vi "10ms loop.vi"(6 "i":i32=12773, 8 "Potent":T2, 9 "Arm Angle":T2={"DevStatus"={"status"=FALSE, "code"=0, "source"=""}, "Analog Module"=enum."Analog Module 1", "Analog Channel"=enum."AI 2"}, 10 "Shooter":T5={"Device"=enum."USB 2"}, 11 "Driver":T5) -> ()   [LabVIEW 2012]
uses:
  <vilib>/Rock Robotics/WPI/AnalogChannel/WPI_AnalogChannelDevRef.ctl
  <vilib>/Rock Robotics/SystemInterfaces/Typedef/FPGA_TypedefAnalogModule.ctl
  <vilib>/Rock Robotics/SystemInterfaces/AI/FPGA_AIChannel.ctl
  <vilib>/Rock Robotics/WPI/Joystick/WPI_JoystickDevRef.ctl
  <vilib>/Rock Robotics/WPI/Joystick/WPI_JoystickDeviceEnum.ctl
  Robot Global Data.vi
panel:
  out "Shooter":T1={"axis 1 (x)"=-0.03937007874015748, "axis 2 (y)"=-0.05511811023622047, "axis 3 (throttle)"=-1.0, "axis 4"=0.0, "axis 5"=0.0, "axis 6"=0.0}
  out "Loop Count":i32=12774
  out "Arm Angle":dbl=1.8048920990000001
  in  "Shooter":dbl(slide)=0.55 min=0.0 max=1.0 step=0.01 scale=0.0..1.0 scale format="%#_2g"
  out "Voltage":dbl=4.728436393
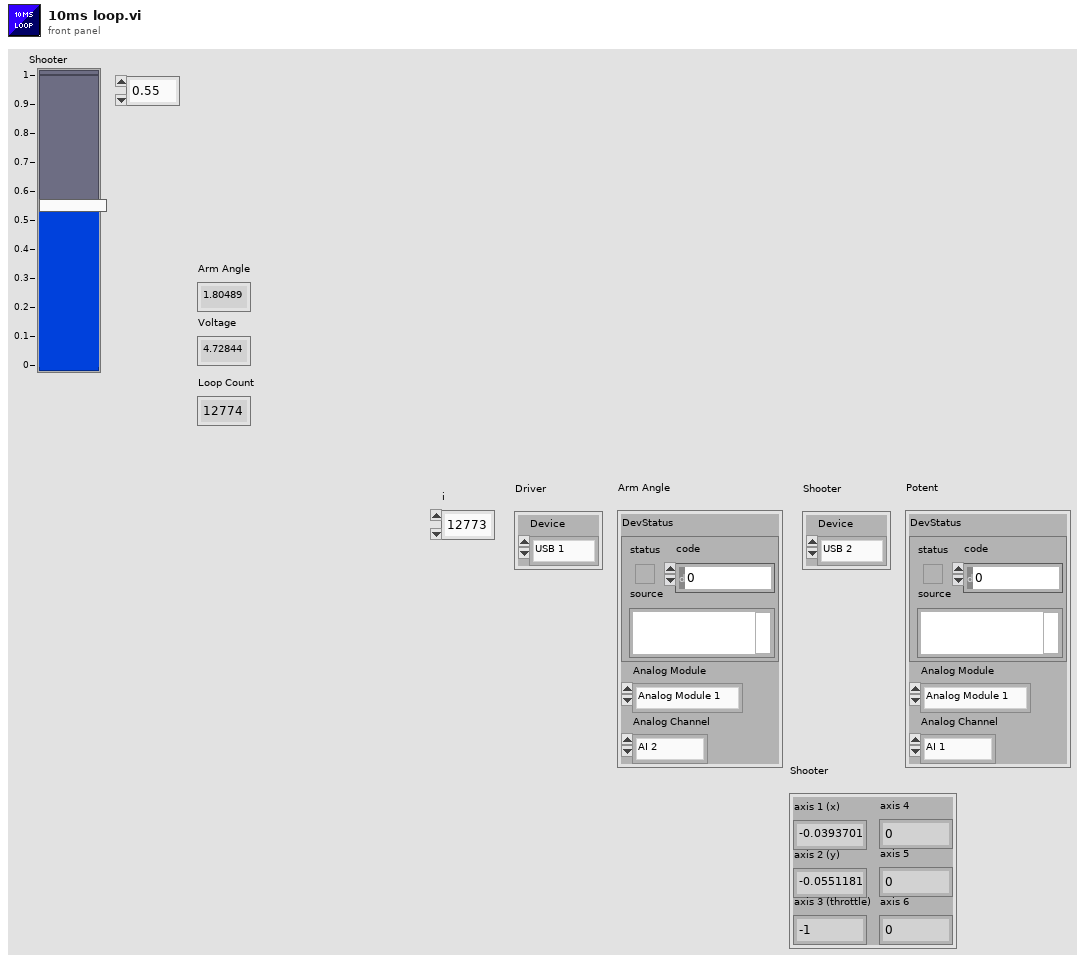
[diagram p1: front panel]
types:
  T1 = cluster{"axis 1 (x)":dbl, "axis 2 (y)":dbl, "axis 3 (throttle)":dbl, "axis 4":dbl, "axis 5":dbl, "axis 6":dbl}
  T2 = typedef "WPI_AnalogChannelDevRef.ctl" = cluster{"DevStatus":errorcluster, "Analog Module":T3, "Analog Channel":T4}
  T3 = typedef "FPGA_TypedefAnalogModule.ctl" = enum16{"Analog Module 1", "Analog Module 2"}
  T4 = typedef "FPGA_AIChannel.ctl" = enum8{"AI 1", "AI 2", "AI 3", "AI 4", "AI 5", "AI 6", "AI 7", "AI 8", "Invalid"}
  T5 = typedef "WPI_JoystickDevRef.ctl" = cluster{"Device":T6}
  T6 = typedef "WPI_JoystickDeviceEnum.ctl" = enum16{"USB 1", "USB 2", "USB 3", "USB 4", "Kinect 1", "Kinect 2"}
  T7 = typedef "WPI_JoystickButtonState.ctl" = cluster{"Button 1":bool, "Button 2":bool, "Button 3":bool, "Button 4":bool, "Button 5":bool, "Button 6":bool, "Button 7":bool, "Button 8":bool, "Button 9":bool, "Button 10":bool, "Button 11":bool, "Button 12":bool}
  T8 = cluster{"Button 6":bool, "Button 7":bool, "Button 11":bool, "Button 10":bool, "Button 2":bool, "Button 3":bool, "Button 1":bool, "Button 4":bool}
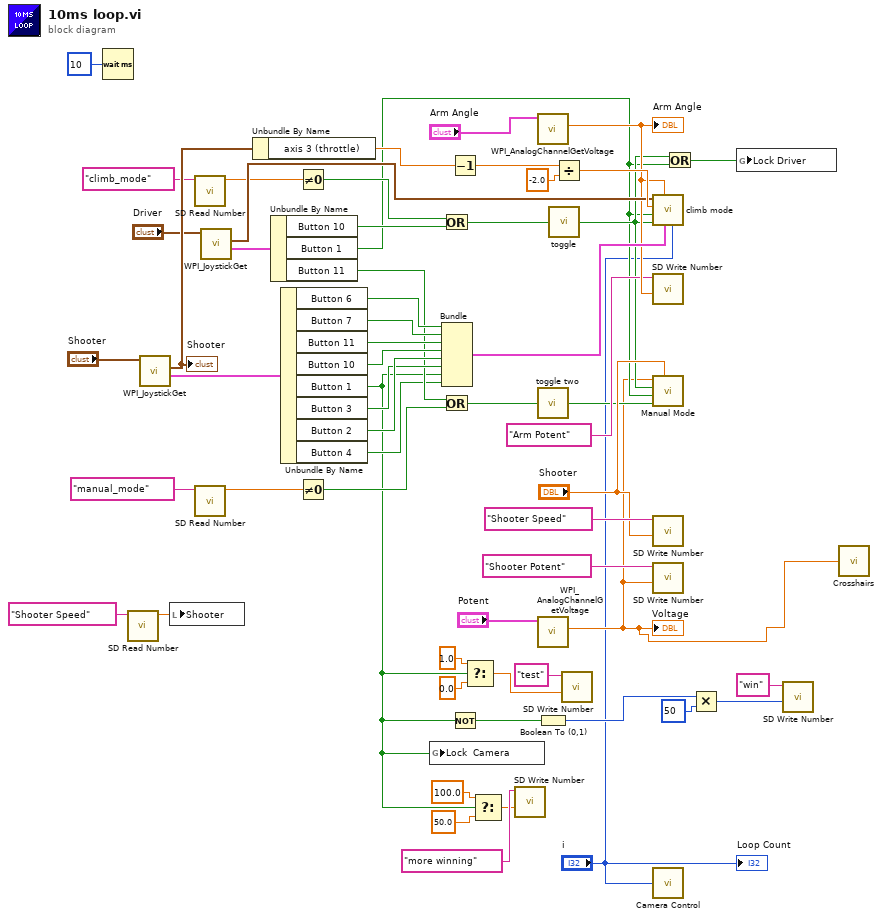
[diagram p0: block diagram]
diagram:
  n1 = Wait (ms)(milliseconds to wait=u32 10) -> ()  [unwired: 1 out]
  n2 = call <vilib>:"SD Read Number.vi"("Name"="Shooter Speed") -> ("Numeric"=w2:dbl)  [unwired: 8 in, 2 out]
  n3 = call <vilib>:"WPI_JoystickGet.vi"("JoystickDevRef"="Shooter") -> ("Buttons"=w56:T7, "Axes"=w50:T1)  [unwired: 4 in, 1 out]
  "Shooter" <- w50
  n4 = local write "Shooter"(w2) -> ()
  n5 = call <vilib>:"SD Read Number.vi"("Name"="climb_mode") -> ("Numeric"=w33:dbl)  [unwired: 8 in, 2 out]
  n6 = call <vilib>:"SD Read Number.vi"("Name"="manual_mode") -> ("Numeric"=w32:dbl)  [unwired: 8 in, 2 out]
  n7 = call <vilib>:"WPI_JoystickGet.vi"("JoystickDevRef"="Driver") -> ("Buttons"=w57:T7, "Axes"=w43:T1)  [unwired: 4 in, 1 out]
  n8 = Unbundle By Name(w50) -> ("axis 3 (throttle)"=w47:dbl)
  n9 = Unbundle By Name(w57) -> ("Button 10"=w29:bool, "Button 1"=w5:bool, "Button 11"=w26:bool)
  n10 = Unbundle By Name(w56) -> ("Button 6"=w54:bool, "Button 7"=w53:bool, "Button 11"=w52:bool, "Button 10"=w51:bool, "Button 1"=w11:bool, "Button 3"=w45:bool, "Button 2"=w46:bool, "Button 4"=w20:bool)
  n11 = Not Equal To 0?(x=w33) -> (x != 0?=w34:bool)
  n12 = Not Equal To 0?(x=w32) -> (x != 0?=w27:bool)
  n13 = global write "Robot Global Data.vi" "Lock  Camera"(w11) -> ()
  n14 = Or(x=w34, y=w29) -> (x .or. y?=w28:bool)
  n15 = Bundle("Button 6"=w54, "Button 7"=w53, "Button 11"=w52, "Button 10"=w51, "Button 2"=w46, "Button 3"=w45, "Button 1"=w11, "Button 4"=w20) -> (w19:T8)  [unwired: 1 in]
  n16 = Or(x=w26, y=w27) -> (x .or. y?=w25:bool)
  n17 = Decrement(x=w47) -> (x-1=w48:dbl)
  n18 = Not(x=w11) -> (.not. x?=w39:bool)
  n19 = Select(t=1.0, s=w11, f=0.0) -> (s? t:f=w23:dbl)
  n20 = Select(t=100.0, s=w11, f=50.0) -> (s? t:f=w12:dbl)
  n21 = call <vilib>:"SD Write Number.vi"("Numeric"=w12, "Name"="more winning") -> ()  [unwired: 8 in, 2 out]
  n22 = call <vilib>:"WPI_AnalogChannelGetVoltage.vi"("AIDeviceRef"="Arm Angle") -> ("Voltage"=w16:dbl)  [unwired: 8 in, 2 out]
  "Arm Angle" <- w16
  n23 = call "toggle two.vi"("Button In"=w25) -> ("tggle Out"=w6:bool)
  n24 = call <vilib>:"WPI_AnalogChannelGetVoltage.vi"("AIDeviceRef"="Potent") -> ("Voltage"=w4:dbl)  [unwired: 8 in, 2 out]
  "Voltage" <- w4
  n25 = Boolean To (0,1)(Boolean=w39) -> (0, 1=w13:i16)
  n26 = call "toggle.vi"("Btn In"=w28) -> ("Toggle Out"=w7:bool)
  n27 = Divide(x=w48, y=-2.0) -> (x/y=w44:dbl)
  n28 = call <vilib>:"SD Write Number.vi"("Numeric"=w23, "Name"="test") -> ()  [unwired: 8 in, 2 out]
  n29 = call "climb mode.vi"("i"="i", "Joystick 2"=w19, "Arm Angle"=w16, "engage climb"=w7, "Button 1"=w5, "Slide"=w44, "Joystick 1 Axes"=w43) -> ()  [unwired: 5 in]
  n30 = call <vilib>:"SD Write Number.vi"("Numeric"=w16, "Name"="Arm Potent") -> ()  [unwired: 8 in, 2 out]
  n31 = call "Manual Mode.vi"("potent"=w4, "Shooter"="Shooter", "climb"=w7, "Button 1"=w5, "manual"=w6) -> ()  [unwired: 4 in]
  n32 = call <vilib>:"SD Write Number.vi"("Numeric"="Shooter", "Name"="Shooter Speed") -> ()  [unwired: 8 in, 2 out]
  n33 = call <vilib>:"SD Write Number.vi"("Numeric"=w4, "Name"="Shooter Potent") -> ()  [unwired: 8 in, 2 out]
  n34 = call "Camera Control.vi"("i"="i") -> ()  [unwired: 1 in]
  n35 = Or(x=w7, y=w5) -> (x .or. y?=w55:bool)
  n36 = Multiply(x=w13, y=i16 50) -> (x*y=w41:i16)
  n37 = global write "Robot Global Data.vi" "Lock Driver"(w55) -> ()
  n38 = call <vilib>:"SD Write Number.vi"("Numeric"=w41, "Name"="win") -> ()  [unwired: 8 in, 2 out]
  n39 = call "Crosshairs.vi"("Potent"=w4) -> ()  [unwired: 1 in]
  "Loop Count" <- "i"
